vi "Complex Conjugate Transpose Matrix.vi"(11 "Input Matrix":T1) -> (0 "error":i32, 3 "Matrix Conjugate Transpose":T1)   [LabVIEW 2020, in "NI_AALPro.lvlib"]
doc: "Transposes <B>Input Matrix</B>. If <B>Input Matrix</B> is a complex matrix, the VI performs conjugate transposition. Wire data to the <B>Input Matrix</B> input to determine the polymorphic instance to use or manually select the instance."
uses:
  NI_AALPro.lvlib
  ComplexMatrix.ctl
  <resource>/lvanlys.dll
  NI_Matrix.lvlib
panel:
  # "Complex  Conjugate Transpose Matrix"
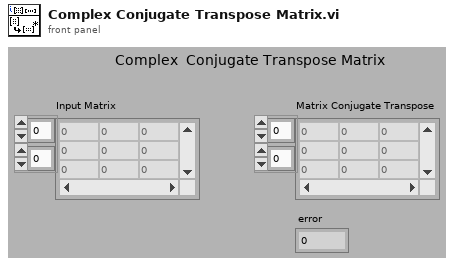
[diagram p1: front panel]
types:
  T1 = typedef "NI_Matrix.lvlib/ComplexMatrix.ctl" = cdb[][]
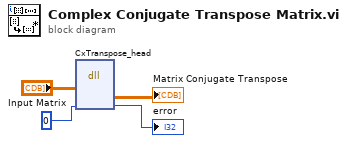
[diagram p0: block diagram]
diagram:
  n1 = dll-call lib="C:/Program Files (x86)/National Instruments/LabVIEW 2020/resource/lvanlys.*" fn="CxTranspose_head"("Input Matrix"="Input Matrix", 0) -> ("Matrix Conjugate Transpose"=→"Matrix Conjugate Transpose":T1, →"error":i32)  [unwired: 6 in, 2 out]
